vi "Get Camera Object.vi"() -> (0 "error out":errorcluster, 3 "Camera out":refnum<class "Camera.lvclass">)   [LabVIEW 2020, in "Camera.lvclass"]
uses:
  Camera.lvclass
  Edmund Optics/Edmund Optics.lvclass
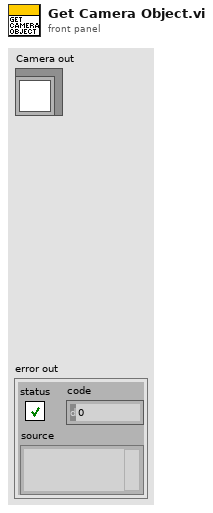
[diagram p1: front panel]
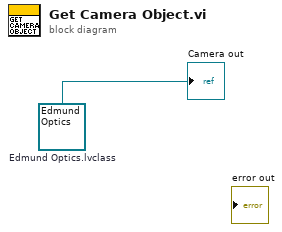
[diagram p0: block diagram]
diagram:
  w1 = refnum<class "Edmund Optics.lvclass"> refnum  # Edmund Optics.lvclass
  "Camera out" <- w1
